vi "Create Volatus API.vi"(8 "error in (no error)":errorcluster, 11 "VolatusCore in":refnum<class "VolatusCoreTask.lvclass">) -> (0 "error out":errorcluster, 3 "VolatusCore out":refnum<class "VolatusCoreTask.lvclass">)   [LabVIEW 2020, in "Volatus.lvlib" / "VolatusCoreTask.lvclass"]
uses:
  VolatusCoreTask.lvclass
  C:/Program Files (x86)/National Instruments/LabVIEW 2020/vi.lib/ActorFramework/Actor/Actor.lvclass
  <vilib>/ActorFramework/Actor/Actor.lvclass/Actor.ctl
  <vilib>/ActorFramework/Message Enqueuer/Message Enqueuer.lvclass/Message Enqueuer.ctl
  VolatusCoreTask.lvclass/VolatusCoreTask.ctl
  <vilib>/ActorFramework/Message Enqueuer/Init from Existing Queue.vi
  VolatusAPI/VolatusAPI.lvclass
  C:/dev/lv20CE/relink/lv-volatus/Volatus/API/API.lvclass
  <vilib>/ActorFramework/Message Enqueuer/Message Enqueuer.lvclass
  <vilib>/ActorFramework/Actor/Actor.lvclass
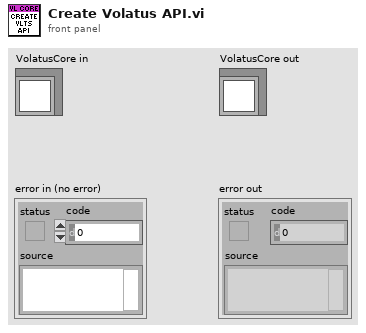
[diagram p1: front panel]
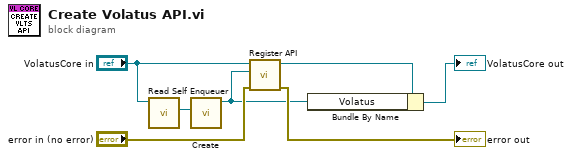
[diagram p0: block diagram]
diagram:
  n1 = call <vilib>:"Read Self Enqueuer.vi"("Actor"="VolatusCore in") -> ("Self Enqueuer"=w6:refnum<class "Message Enqueuer.lvclass">)  [unwired: 10 in]
  n2 = call "Create.vi"("EnQr"=w6) -> ("VolatusAPI out"=w1:refnum<class "VolatusAPI.lvclass">)  [unwired: 9 in, 1 out]
  n3 = call-dynamic "Register API.vi"("error in (no error)"="error in (no error)", "API"=w1, "VolatusCore in"="VolatusCore in") -> ("error out"=→"error out":errorcluster, "VolatusCore out"=w5:refnum<class "VolatusCoreTask.lvclass">)  [unwired: 7 in]
  n4 = Bundle By Name(cluster=w5, "Volatus"=w1) -> (→"VolatusCore out":refnum<class "VolatusCoreTask.lvclass">)
